vi "ClimbExecute.vi"(8 "error in (no error)":errorcluster) -> (0 "error out":errorcluster)   [LabVIEW 2023]
uses:
  <vilib>/Rock Robotics/WPI/ThirdParty/JAS_Junk/TrajLib/Trajectory_Library.lvlib
  ClimbNetworkingGlobal.vi
  <vilib>/Rock Robotics/WPI/ThirdParty/REV Robotics/REVLib/SubVI/Public/SPARK Get Limit Switch Status Reverse.vi
  <vilib>/Rock Robotics/WPI/ThirdParty/REV Robotics/REVLib/SubVI/Public/SPARK Get Encoder Status Position.vi
  <vilib>/Rock Robotics/WPI/ThirdParty/REV Robotics/REVLib/Typedef/Spark MAX Control Type.ctl
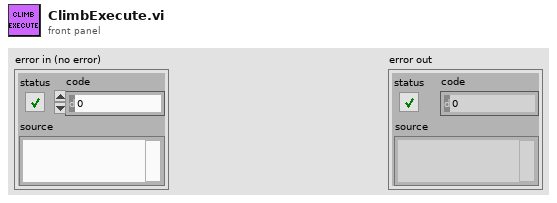
[diagram p1: front panel]
types:
  T1 = typedef "Spark MAX Control Type.ctl" = enum16{"Percent VBus", "Voltage", "Velocity", "Position", "Smart Motion", "Current", "Smart Velocity", "MAXMotion Position", "MAXMotion Velocity"}
  T2 = typedef "WPI_MotorControlDeviceRef.ctl" = cluster{"DeviceStatus":errorcluster, "Type":T3, "PWM":cluster{"PWM Channel":T4, "DeadBand":T5}, "CAN":cluster{"Device Number":u8, "SetOutput VI Ref":variant, "GetOutput VI Ref":variant, "Enable VI Ref":variant, "Disable VI Ref":variant, "Data":variant}, "Invert":bool, "DIO PWM":cluster{"PWM \"Enable\" Channel":T4, "DIOChannel":T6, "PWM Rate":dbl}}
  T3 = typedef "WPI_MotorControlType.ctl" = enum16{"PWM", "CAN", "DIO PWM"}
  T4 = typedef "FPGA_DIOPWMChannel.ctl" = enum8{"PWM 0", "PWM 1", "PWM 2", "PWM 3", "PWM 4", "PWM 5", "PWM 6", "PWM 7", "PWM 8", "PWM 9", "PWM MXP 0", "PWM MXP 1", "PWM MXP 2", "PWM MXP 3", "PWM MXP 4", "PWM MXP 5", "PWM MXP 6", "PWM MXP 7", "PWM MXP 8", "PWM MXP 9", "Invalid"}
  T5 = typedef "WPI_PWMDeadband.ctl" = cluster{"Name":string, "maxPositivePwm":i32, "minPositivePwm":i32, "centerPwm":i32, "maxNegativePwm":i32, "minNegativePwm":i32, "angularRange":u16}
  T6 = typedef "FPGA_DIOChannel.ctl" = enum8{"DIO 0", "DIO 1", "DIO 2", "DIO 3", "DIO 4", "DIO 5", "DIO 6", "DIO 7", "DIO 8", "DIO 9", "DIO MXP 0", "DIO MXP 1", "DIO MXP 2", "DIO MXP 3", "DIO MXP 4", "DIO MXP 5", "DIO MXP 6", "DIO MXP 7", "DIO MXP 8", "DIO MXP 9", "DIO MXP 10", "DIO MXP 11", "DIO MXP 12", "DIO MXP 13", "DIO MXP 14", "DIO MXP 15", "SPI Port CS1", "SPI Port CS2", "SPI Port CS3", "SPI Port MISO", "SPI Port MOSI", "Invalid"}
  T7 = typedef "Trajectory_Library.lvlib/PosCtrl_Tuning_Type.ctl" = cluster{"Slope":dbl, "Offset":dbl, "Error Deadband":dbl, "At Reference Count":i32, "Negate Output":bool, "Max Allowd Position":dbl, "Min Allowd Position":dbl}
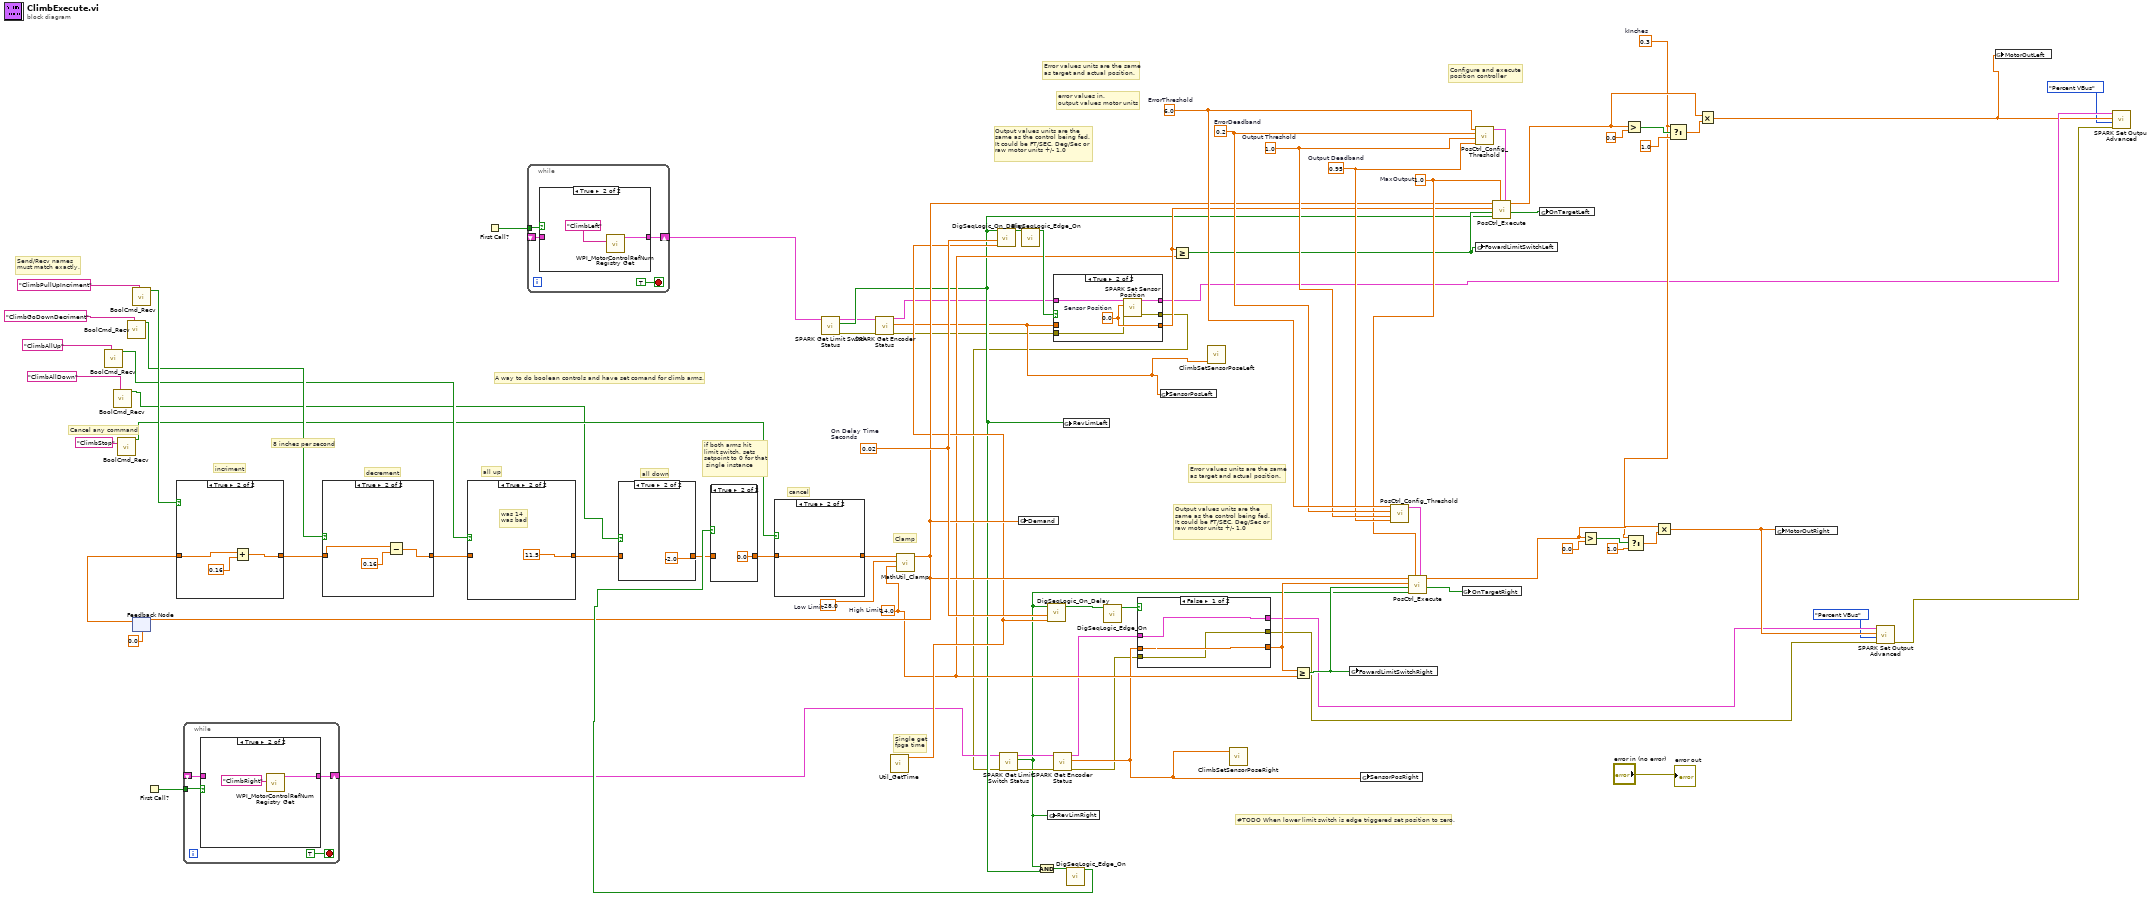
[diagram p0: block diagram]
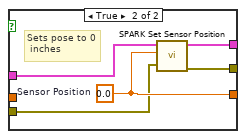
[diagram p6: hidden frame]
diagram:
  w24 = 14.0  # High Limit
  w38 = 0.3  # kInches
  w52 = 0.02  # On Delay Time Seconds
  w67 = -28.0  # Low Limit
  w54 = 1.0  # MaxOutput
  w58 = 6.0  # ErrorThreshold
  w57 = 0.2  # ErrorDeadband
  w56 = 1.0  # Output Threshold
  w55 = 0.95  # Output Deadband
  # "Single get\nfpga time"
  # "if both arms hit \nlimit switch, sets \nsetpoint to 0 for that\n single instance"
  # "#TODO When lower limit switch is edge triggered set position to zero."
  # "cancel"
  # "Clamp"
  # "8 inches per second"
  # "all down"
  # "all up"
  # "decrement"
  # "incriment"
  # "Cancel any command"
  # "Send/Recv names\nmust match exactly."
  # "A way to do boolean controls and have set comand for climb arms."
  # "error values in.\noutput values motor units"
  # "Output values units are the\nsame as the control being fed.  \nIt could be FT/SEC, Deg/Sec or\nraw motor units +/- 1.0"
  # "Error values units are the same \nas target and actual position."
  # "Output values units are the\nsame as the control being fed.  \nIt could be FT/SEC, Deg/Sec or\nraw motor units +/- 1.0"
  # "Error values units are the same \nas target and actual position."
  # "Configure and execute \nposition controller"
  n1 = call <vilib>:"BoolCmd_Recv.vi"("Command Name"="ClimbAllUp") -> ("New Request"=w63:bool)  [unwired: 9 in, 1 out]
  n2 = call <vilib>:"BoolCmd_Recv.vi"("Command Name"="ClimbAllDown") -> ("New Request"=w35:bool)  [unwired: 9 in, 1 out]
  n3 = call <vilib>:"BoolCmd_Recv.vi"("Command Name"="ClimbStop") -> ("New Request"=w62:bool)  [unwired: 9 in, 1 out]
  n4 = call <vilib>:"BoolCmd_Recv.vi"("Command Name"="ClimbGoDownDecriment") -> ("New Request"=w64:bool)  [unwired: 9 in, 1 out]
  n5 = call <vilib>:"BoolCmd_Recv.vi"("Command Name"="ClimbPullUpIncriment") -> ("New Request"=w65:bool)  [unwired: 9 in, 1 out]
  n6 = feedback #1(0.0 ("false")) -> (w71:dbl)
  n7 = First Call?() -> (First Call?: T/F=w32:bool)
  n8 = case shown="True" w65 {
    tunnel: w71 -> [w80 w83]
    tunnel: [w80 w81] -> w70
    frame False {
    }
    frame True {
      n9 = Add(x=w83, y=0.16) -> (x+y=w81:dbl)
    }
  }
  n10 = while {
    tunnel: w32 -> [w86]
    shift-right: [w87] -> w14
    shift-left: _ -> [w85]
    stop <- TRUE stop-if-true
    n11 = case shown="True" w86 {
      tunnel: [w88 w90] -> w87
      tunnel: w85 -> [w88 _]
      frame False {
      }
      frame True {
        n12 = call <vilib>:"WPI_MotorControlRefNum Registry Get.vi"("refnum name"="ClimbRight") -> ("MotorControlDevRef"=w90:T2)  [unwired: 9 in, 1 out]
      }
    }
  }
  n13 = case shown="True" w64 {
    tunnel: w70 -> [w91 w93]
    tunnel: [w91 w92] -> w69
    frame False {
    }
    frame True {
      n14 = Subtract(x=w93, y=0.16) -> (x-y=w92:dbl)
    }
  }
  n15 = case shown="True" w63 {
    tunnel: w69 -> [w95 _]
    tunnel: [w95 11.5 ("y")] -> w68
    frame False {
    }
    frame True {
      # "was 14\nwas bad"
    }
  }
  n16 = First Call?() -> (First Call?: T/F=w31:bool)
  n17 = while {
    tunnel: w31 -> [w99]
    shift-right: [w100] -> w23
    shift-left: _ -> [w98]
    stop <- TRUE stop-if-true
    n18 = case shown="True" w99 {
      tunnel: [w101 w103] -> w100
      tunnel: w98 -> [w101 _]
      frame False {
      }
      frame True {
        n19 = call <vilib>:"WPI_MotorControlRefNum Registry Get.vi"("refnum name"="ClimbLeft") -> ("MotorControlDevRef"=w103:T2)  [unwired: 9 in, 1 out]
      }
    }
  }
  n20 = case shown="True" w35 {
    tunnel: w68 -> [w104 _]
    tunnel: [w104 -2.0 ("y")] -> w34
    frame False {
    }
    frame True {
    }
  }
  n21 = call-poly <vilib>:"SPARK Get Limit Switch Status.vi"("MotorControlDevRef in"=w23) -> ("error out"=w20:errorcluster, "Hard Limit Rev"=w22:bool, "MotorControlDevRef out"=w21:T2)  [unwired: 7 in, 1 out]
  n22 = call-poly <vilib>:"SPARK Get Encoder Status.vi"("error in (no error)"=w20, "MotorControlDevRef in"=w21) -> ("error out"=w17:errorcluster, "Sensor Position"=w19:dbl, "MotorControlDevRef out"=w18:T2)  [unwired: 6 in, 1 out]
  n23 = call <vilib>:"Util_GetTime.vi"() -> ("FPGA_Time_Seconds"=w25:dbl)  [unwired: 9 in, 2 out]
  n24 = call <vilib>:"DigSeqLogic_On_Delay.vi"("Time"=w25, "Delay"=w52, "Input"=w22) -> ("Output"=w51:bool)  [unwired: 7 in, 1 out]
  n25 = call <vilib>:"DigSeqLogic_Edge_On.vi"("Input"=w51) -> ("On Edge"=w50:bool)  [unwired: 10 in]
  n26 = case shown="True" w50 {
    tunnel: w18 -> [w108 w113]
    tunnel: [w108 w112] -> w4
    tunnel: w19 -> [w107 _]
    tunnel: [w107 w111] -> w49
    tunnel: w17 -> [w106 w110]
    tunnel: [w106 w109] -> w13
    frame False {
    }
    frame True {
      w111 = 0.0  # Sensor Position
      n27 = call <vilib>:"SPARK Set Sensor Position.vi"("error in"=w110, "Position"=w111, "MotorControlDeviceRef"=w113) -> ("error out"=w109:errorcluster, "MotorControlDeviceRef"=w112:T2)  [unwired: 7 in]
    }
  }
  n28 = call-poly <vilib>:"SPARK Get Limit Switch Status.vi"("error in (no error)"=w13, "MotorControlDevRef in"=w14) -> ("error out"=w15:errorcluster, "Hard Limit Rev"=w12:bool, "MotorControlDevRef out"=w16:T2)  [unwired: 6 in, 1 out]
  n29 = And(x=w12, y=w22) -> (x .and. y?=w37:bool)
  n30 = call <vilib>:"DigSeqLogic_On_Delay.vi"("Time"=w25, "Delay"=w52, "Input"=w12) -> ("Output"=w60:bool)  [unwired: 7 in, 1 out]
  n31 = global write "ClimbNetworkingGlobal.vi" "RevLimRight"(w12) -> ()
  n32 = call-poly <vilib>:"SPARK Get Encoder Status.vi"("error in (no error)"=w15, "MotorControlDevRef in"=w16) -> ("error out"=w10:errorcluster, "Sensor Position"=w11:dbl, "MotorControlDevRef out"=w9:T2)  [unwired: 6 in, 1 out]
  n33 = global write "ClimbNetworkingGlobal.vi" "RevLimLeft"(w22) -> ()
  n34 = call <vilib>:"DigSeqLogic_Edge_On.vi"("Input"=w37) -> ("On Edge"=w36:bool)  [unwired: 10 in]
  n35 = case shown="True" w36 {
    tunnel: w34 -> [w114 _]
    tunnel: [w114 0.0 ("y")] -> w33
    frame False {
    }
    frame True {
    }
  }
  n36 = case shown="True" w62 {
    tunnel: w33 -> [w116 w117]
    tunnel: [w116 w117] -> w66
    frame False {
    }
    frame True {
    }
  }
  n37 = call <vilib>:"MathUtil_Clamp.vi"("High Limit"=w24, "Low Limit"=w67, "Value"=w66) -> ("Result"=w26:dbl)  [unwired: 8 in]
  n38 = feedback-in #1(w26) -> ()
  n39 = global write "ClimbNetworkingGlobal.vi" "Demand"(w26) -> ()
  n40 = call <vilib>:"DigSeqLogic_Edge_On.vi"("Input"=w60) -> ("On Edge"=w53:bool)  [unwired: 10 in]
  n41 = case shown="False" w53 {
    tunnel: w11 -> [w120 _]
    tunnel: [w120 w125] -> w59
    tunnel: w10 -> [w119 w124]
    tunnel: [w119 w123] -> w6
    tunnel: w9 -> [w118 w122]
    tunnel: [w118 w121] -> w7
    frame False {
    }
    frame True {
      w125 = 0.0  # Sensor Position
      # "Sets pose to 0\n inches"
      n42 = call <vilib>:"SPARK Set Sensor Position.vi"("error in"=w124, "Position"=w125, "MotorControlDeviceRef"=w122) -> ("error out"=w123:errorcluster, "MotorControlDeviceRef"=w121:T2)  [unwired: 7 in]
    }
  }
  n43 = global write "ClimbNetworkingGlobal.vi" "SensorPosLeft"(w19) -> ()
  n44 = Greater Or Equal?(x=w49, y=w24) -> (x >= y?=w27:bool)
  n45 = call "ClimbSetSensorPoseLeft.vi"("ClimbSetSensorPoseLeft"=w19) -> ()  [unwired: 11 in]
  n46 = call "ClimbSetSensorPoseRight.vi"("ClimbSetSensorPoseRight"=w11) -> ()  [unwired: 11 in]
  n47 = Greater Or Equal?(x=w59, y=w24) -> (x >= y?=w30:bool)
  n48 = global write "ClimbNetworkingGlobal.vi" "FowardLimitSwitchRight"(w30) -> ()
  n49 = global write "ClimbNetworkingGlobal.vi" "SensorPosRight"(w11) -> ()
  n50 = call <vilib>:"PosCtrl_Config_Threshold.vi"("Output Deadband"=w55, "Output Threshold"=w56, "ErrorDeadband"=w57, "ErrorThreshold"=w58) -> ("PosCtrl_Config_Params"=w78:T7)  [unwired: 7 in]
  n51 = call <vilib>:"PosCtrl_Execute.vi"("PosCtrl_Config_Params"=w78, "MaxOutput"=w54, "Rev Limit Switch"=w12, "Fwd Limit Switch"=w30, "CurrentPosition"=w59, "TargetPosition"=w26) -> ("OnTarget"=w29:bool, "Output"=w39:dbl)  [unwired: 3 in, 1 out]
  n52 = global write "ClimbNetworkingGlobal.vi" "OnTargetRight"(w29) -> ()
  n53 = call <vilib>:"PosCtrl_Config_Threshold.vi"("Output Deadband"=w55, "Output Threshold"=w56, "ErrorDeadband"=w57, "ErrorThreshold"=w58) -> ("PosCtrl_Config_Params"=w79:T7)  [unwired: 7 in]
  n54 = global write "ClimbNetworkingGlobal.vi" "FowardLimitSwitchLeft"(w27) -> ()
  n55 = call <vilib>:"PosCtrl_Execute.vi"("PosCtrl_Config_Params"=w79, "MaxOutput"=w54, "Rev Limit Switch"=w22, "Fwd Limit Switch"=w27, "CurrentPosition"=w49, "TargetPosition"=w26) -> ("OnTarget"=w28:bool, "Output"=w44:dbl)  [unwired: 3 in, 1 out]
  n56 = global write "ClimbNetworkingGlobal.vi" "OnTargetLeft"(w28) -> ()
  n57 = Greater?(x=w39, y=0.0) -> (0:w42:bool)
  n58 = Greater?(x=w44, y=0.0) -> (0:w47:bool)
  n59 = Select(t=w38, s=w42, f=1.0) -> (s? t:f=w40:dbl)
  n60 = Multiply(x=w39, y=w40) -> (x*y=w8:dbl)
  n61 = Select(t=w38, s=w47, f=1.0) -> (s? t:f=w45:dbl)
  n62 = Multiply(x=w44, y=w45) -> (x*y=w2:dbl)
  n63 = global write "ClimbNetworkingGlobal.vi" "MotorOutRight"(w8) -> ()
  n64 = call <vilib>:"SPARK Set Output Advanced.vi"("error in (no error)"=w6, "Control Mode"=Spark_MAX_Control_Type."Percent VBus", "Setpoint"=w8, "MotorControlDevRef"=w7) -> ("error out"=w3:errorcluster)  [unwired: 6 in, 1 out]
  n65 = global write "ClimbNetworkingGlobal.vi" "MotorOutLeft"(w2) -> ()
  n66 = call <vilib>:"SPARK Set Output Advanced.vi"("error in (no error)"=w3, "Control Mode"=Spark_MAX_Control_Type."Percent VBus", "Setpoint"=w2, "MotorControlDevRef"=w4) -> ()  [unwired: 6 in, 2 out]
  "error out" <- "error in (no error)"
